vi "DFD M-Band Filter Bank Decomposition.vi"   [LabVIEW 2017, in "NI_DigFilter_FilterBank.lvlib"]
doc: "Decomposes a signal into M-band signals continuously with a cosine-modulated filter bank."
uses:
  <vilib>/addons/Digital Filter Design/NI_DigFilter_FilterBank.lvlib
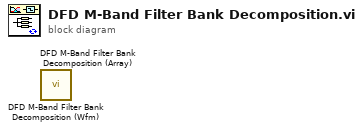
[diagram p0: block diagram]
diagram:
  n1 = call <vilib>:"DFD M-Band Filter Bank Decomposition (Wfm).vi"() -> ()  [unwired: 10 in, 2 out]
  n2 = call <vilib>:"DFD M-Band Filter Bank Decomposition (Array).vi"() -> ()  [unwired: 10 in, 2 out]
